vi "genRtPrbs.vi"(11 "Amplitude":dbl=0.2 format="%#_13g") -> (3 "signal":dbl)   [LabVIEW 2020, in "Communication.lvclass"]
uses:
  Communication.lvclass
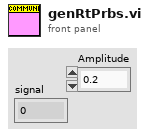
[diagram p1: front panel]
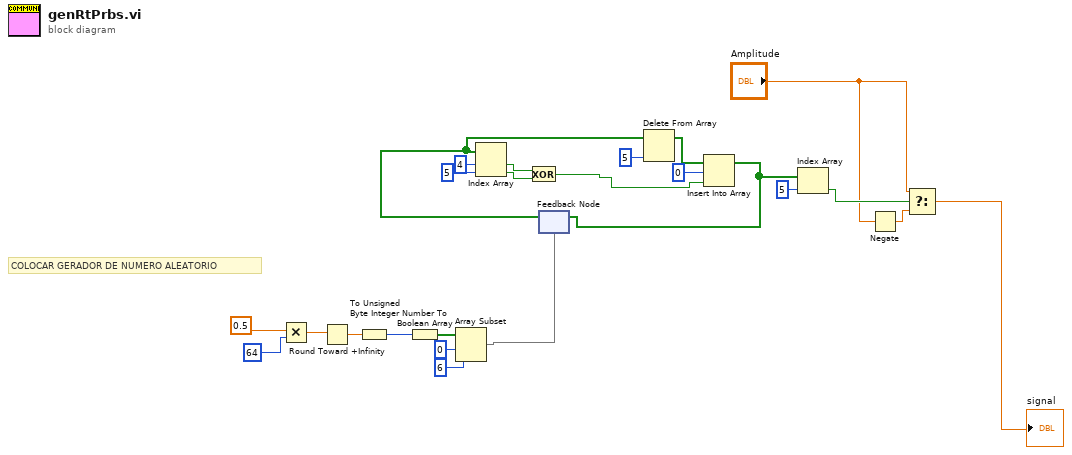
[diagram p0: block diagram]
diagram:
  # "COLOCAR GERADOR DE NUMERO ALEATORIO"
  n1 = Multiply(x=0.5, y=64) -> (x*y=w2:dbl)
  n2 = Round Toward +Infinity(x=w2) -> (ceil(x): smallest int >= x=w4:dbl)
  n3 = To Unsigned Byte Integer(number=w4) -> (unsigned 8bit integer=w5:u8)
  n4 = Number To Boolean Array(number=w5) -> (Boolean array=w6:bool[])
  n5 = Array Subset(array=w6, index=0, length=6) -> (w9:bool[])
  n6 = feedback #1(w9) -> (w10:bool[])
  n7 = Index Array(array=w10, index #1=4 ("index"), index #2=5 ("index")) -> (element #1=w15:bool, element #2=w16:bool)
  n8 = Exclusive Or(1:w16, 2:w15) -> (0:w23:bool)
  n9 = Delete From Array(array=w10, index=5) -> (array with subset deleted=w18:bool[])  [unwired: 1 in, 1 out]
  n10 = Insert Into Array(array=w18, index=0, new element=w23) -> (w20:bool[])
  n11 = feedback-in #1(w20) -> ()
  n12 = Index Array(array=w20, index=5) -> (element=w22:bool)
  n13 = Negate(x="Amplitude") -> (-x=w11:dbl)
  n14 = Select(t="Amplitude", s=w22, f=w11) -> (s? t:f=→"signal":dbl)
